vi "ILM_Merge_Cluster.vi"(1 "SR830-2 3":T2, 2 "SR830-2 4":T1 {"Nitrogen" format="%#4_5f"}) -> (0 "SR830-2 2":T3 {"Nitrogen" format="%#4_5f"})   [LabVIEW 2019]
uses:
  S16/ILM-Cluster.ctl
  S16/ILM-Control.ctl
  S16/ILM-Status.ctl
panel:
  # "N (%)"
  # "He (%)"
  # "Levelmeter"
  # "N (%)"
  # "He (%)"
  # "Levelmeter"
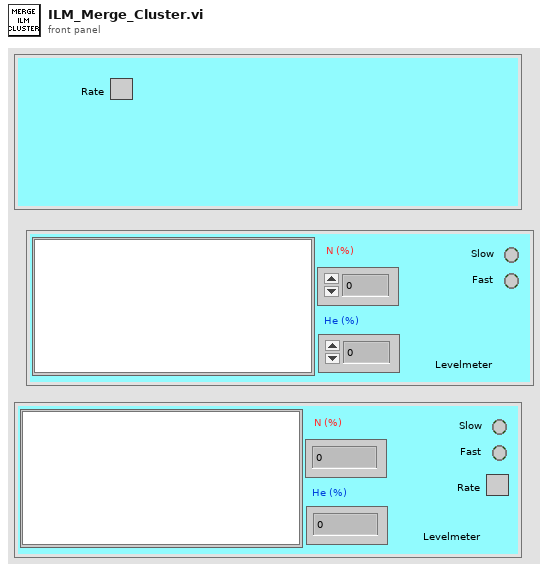
[diagram p1: front panel]
types:
  T1 = typedef "ILM-Status.ctl" = cluster{"Plot":dbl[][], "Nitrogen":dbl, "Helium":dbl, "Fast":bool, "Slow":bool}
  T2 = typedef "ILM-Control.ctl" = cluster{"Rate":bool}
  T3 = typedef "ILM-Cluster.ctl" = cluster{"Plot":dbl[][], "Nitrogen":dbl, "Helium":dbl, "Fast":bool, "Slow":bool, "Rate":bool}
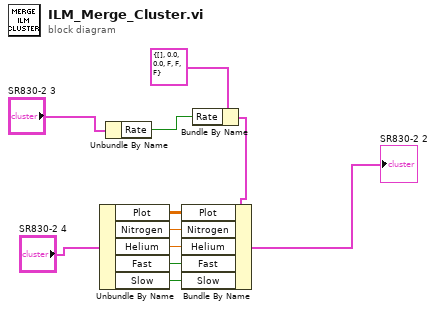
[diagram p0: block diagram]
diagram:
  n1 = Unbundle By Name("SR830-2 4") -> ("Plot"=w11:dbl[][], "Nitrogen"=w10:dbl, "Helium"=w9:dbl, "Fast"=w8:bool, "Slow"=w7:bool)
  n2 = Unbundle By Name("SR830-2 3") -> ("Rate"=w6:bool)
  n3 = Bundle By Name(cluster=T3 {"Plot"=[], "Nitrogen"=0.0, "Helium"=0.0, "Fast"=FALSE, "Slow"=FALSE, "Rate"=FALSE} ("SR830-2 5"), "Rate"=w6) -> (w4:T3)
  n4 = Bundle By Name(cluster=w4, "Plot"=w11, "Nitrogen"=w10, "Helium"=w9, "Fast"=w8, "Slow"=w7) -> (→"SR830-2 2":T3)
